vi "986x.Export.vi"(8 "error in (no error)":errorcluster, 11 "Device Item Ref in":T2 format="%.0x") -> (0 "error out":errorcluster, 2 "986x Support":T1, 3 "Item Ref out":T2 format="%.0x")   [LabVIEW 2020, in "Protection and Counter Addon System Explorer.lvlib"]
uses:
  Protection and Counter Addon System Explorer.lvlib
  <vilib>/NI VeriStand/Custom Device API/Custom Device Item Ref.ctl
  Addon Shared/Types/986x.ctl
  Addon Shared/SubVIs/GUID Lookup.vi
  <vilib>/NI VeriStand/Custom Device API/Get Item Property (Boolean).vi
  <vilib>/NI VeriStand/Custom Device API/Get Item Property (String).vi
  <vilib>/NI VeriStand/Custom Device API/Get Item Property (Dependent File).vi
  <vilib>/NI VeriStand/Custom Device API/Get Item Property (U32).vi
  <vilib>/NI VeriStand/Custom Device API/Get Item Property (String Array).vi
  <vilib>/NI VeriStand/Custom Device API/Custom Device API.lvlib
  Addon Shared/Protection and Counter Addon Shared.lvlib
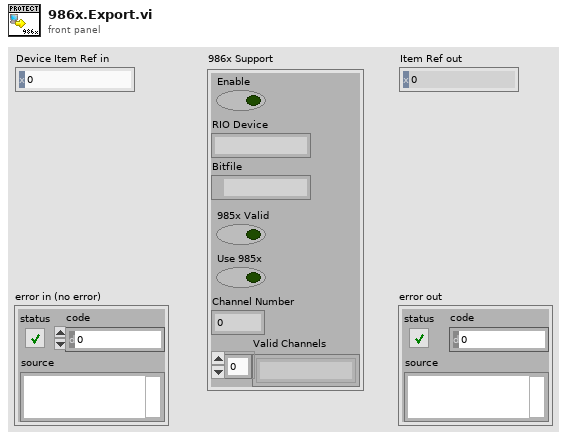
[diagram p1: front panel]
types:
  T1 = typedef "Protection and Counter Addon Shared.lvlib/986x.ctl" = cluster{"Enable":bool, "RIO Device":string, "Bitfile":path, "985x Valid":bool, "Use 985x":bool, "Channel Number":u32, "Valid Channels":string[]}
  T2 = typedef "Custom Device API.lvlib/Custom Device Item Ref.ctl" = u64
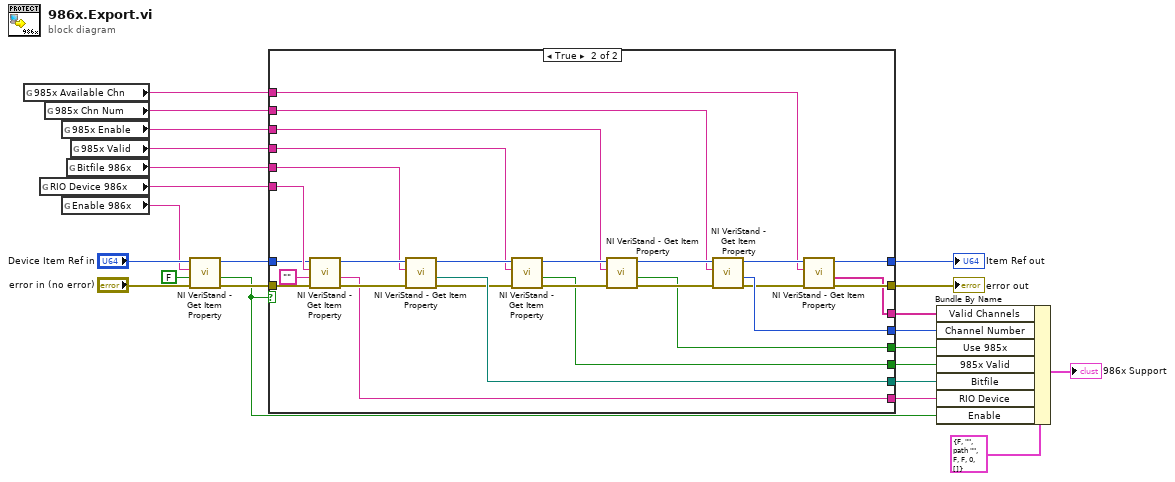
[diagram p0: block diagram]
diagram:
  n1 = global read "GUID Lookup.vi" "985x Available Chn"() -> (w2:string)
  n2 = global read "GUID Lookup.vi" "RIO Device 986x"() -> (w10:string)
  n3 = global read "GUID Lookup.vi" "985x Chn Num"() -> (w4:string)
  n4 = global read "GUID Lookup.vi" "985x Enable"() -> (w6:string)
  n5 = global read "GUID Lookup.vi" "Enable 986x"() -> (w11:string)
  n6 = global read "GUID Lookup.vi" "Bitfile 986x"() -> (w9:string)
  n7 = global read "GUID Lookup.vi" "985x Valid"() -> (w8:string)
  n8 = call-poly <vilib>:"NI VeriStand - Get Item Property.vi"("error in (no error)"="error in (no error)", "Default Value"=FALSE, "Property Name"=w11, "Item Ref in"="Device Item Ref in") -> ("error out"=w20:errorcluster, "Value"=w15:bool, "Item Ref out"=w21:T2)  [unwired: 4 in, 1 out]
  n9 = case shown="True" w15 {
    tunnel: w20 -> [w25 w52]
    tunnel: [w25 w27] -> w22
    tunnel: w10 -> [_ w51]
    tunnel: w9 -> [_ w48]
    tunnel: w21 -> [w24 w47]
    tunnel: [w24 w30] -> w23
    tunnel: [_ w46] -> w13
    tunnel: [_ w45] -> w14
    tunnel: w8 -> [_ w37]
    tunnel: [_ w36] -> w7
    tunnel: w6 -> [_ w35]
    tunnel: [_ w34] -> w5
    tunnel: w4 -> [_ w33]
    tunnel: [_ w32] -> w3
    tunnel: w2 -> [_ w28]
    tunnel: [_ w26] -> w1
    frame False {
    }
    frame True {
      n10 = call-poly <vilib>:"NI VeriStand - Get Item Property.vi"("error in (no error)"=w52, "Default Value"="", "Property Name"=w51, "Item Ref in"=w47) -> ("error out"=w50:errorcluster, "Value"=w46:string, "Item Ref out"=w49:T2)  [unwired: 4 in, 1 out]
      n11 = call-poly <vilib>:"NI VeriStand - Get Item Property.vi"("error in (no error)"=w50, "Property Name"=w48, "Item Ref in"=w49) -> ("error out"=w38:errorcluster, "Path"=w45:path, "Item Ref out"=w43:T2)  [unwired: 4 in, 2 out]
      n12 = call-poly <vilib>:"NI VeriStand - Get Item Property.vi"("error in (no error)"=w38, "Property Name"=w37, "Item Ref in"=w43) -> ("error out"=w41:errorcluster, "Value"=w36:bool, "Item Ref out"=w42:T2)  [unwired: 5 in, 1 out]
      n13 = call-poly <vilib>:"NI VeriStand - Get Item Property.vi"("error in (no error)"=w41, "Property Name"=w35, "Item Ref in"=w42) -> ("error out"=w39:errorcluster, "Value"=w34:bool, "Item Ref out"=w40:T2)  [unwired: 5 in, 1 out]
      n14 = call-poly <vilib>:"NI VeriStand - Get Item Property.vi"("error in (no error)"=w39, "Property Name"=w33, "Item Ref in"=w40) -> ("error out"=w29:errorcluster, "Value"=w32:u32, "Item Ref out"=w31:T2)  [unwired: 5 in, 1 out]
      n15 = call-poly <vilib>:"NI VeriStand - Get Item Property.vi"("error in (no error)"=w29, "Property Name"=w28, "Item Ref in"=w31) -> ("error out"=w27:errorcluster, "Value"=w26:string[], "Item Ref out"=w30:T2)  [unwired: 5 in, 1 out]
    }
  }
  "Item Ref out" <- w23
  "error out" <- w22
  n16 = Bundle By Name(cluster=T1 {"Enable"=FALSE, "RIO Device"="", "Bitfile"=path "", "985x Valid"=FALSE, "Use 985x"=FALSE, "Channel Number"=0, "Valid Channels"=[]}, "Valid Channels"=w1, "Channel Number"=w3, "Use 985x"=w5, "985x Valid"=w7, "Bitfile"=w14, "RIO Device"=w13, "Enable"=w15) -> (→"986x Support":T1)
